vi "HB_OpenLog.vi"(8 "error in (no error)":errorcluster, 10 "File Name":string, 11 "“HBDeviceRef_in":T1) -> (0 "error out":errorcluster, 3 "“HBDeviceRef_out":T1)   [LabVIEW 2016]
uses:
  <vilib>/Rock Robotics/WPI/SerialPort/WPI_SerialPortRef.ctl
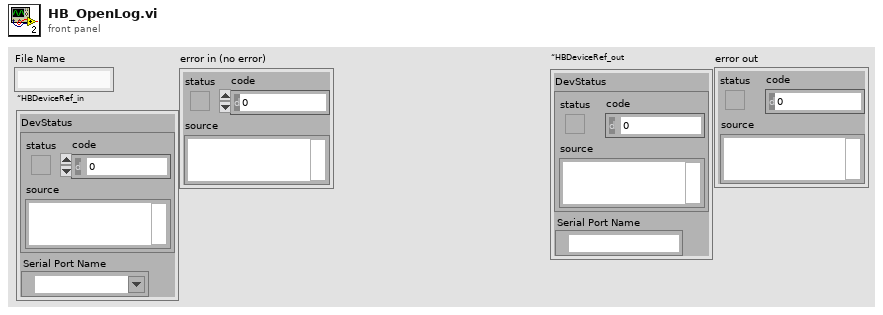
[diagram p1: front panel]
types:
  T1 = typedef "WPI_SerialPortRef.ctl" = cluster{"DevStatus":errorcluster, "Serial Port Name":refnum<visa-resource-name>}
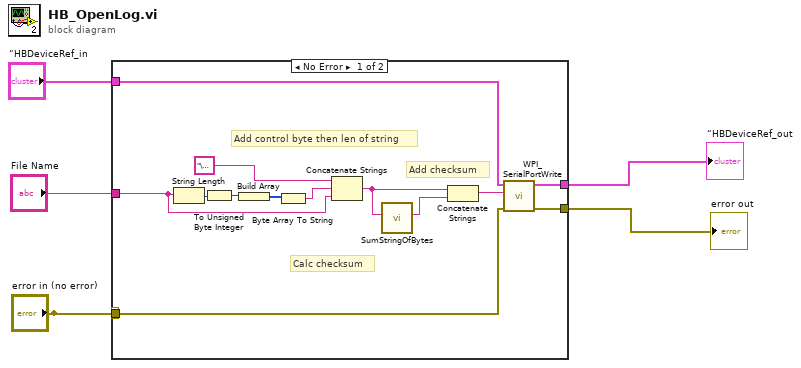
[diagram p0: block diagram]
diagram:
  n1 = case shown="No Error" "error in (no error)" {
    selector: "error in (no error)" -> [_ w19]
    tunnel: "File Name" -> [w10 _]
    tunnel: "“HBDeviceRef_in" -> [w9 w20]
    tunnel: [w8 w20] -> w3
    tunnel: "error in (no error)" -> [w7 _]
    tunnel: [w6 w19] -> w2
    frame No Error {
      # "Calc checksum"
      # "Add checksum"
      # "Add control byte then len of string"
      n2 = String Length(string=w10) -> (length=w12:i32)
      n3 = To Unsigned Byte Integer(number=w12) -> (unsigned 8bit integer=w15:u8)
      n4 = Build Array(w15) -> (w14:u8[])
      n5 = Byte Array To String(unsigned byte array=w14) -> (string=w13:string)
      n6 = Concatenate Strings("\u0003", w13, w10) -> (w17:string)
      n7 = call "SumStringOfBytes.vi"("String Of Bytes"=w17) -> ("SumAsString"=w18:string)  [unwired: 10 in]
      n8 = Concatenate Strings(w17, w18) -> (w11:string)
      n9 = call <vilib>:"WPI_SerialPortWrite.vi"("error in (no error)"=w7, "Buffer"=w11, "SerialPortRef"=w9) -> ("error out"=w6:errorcluster, "SerialPortRef"=w8:T1)  [unwired: 6 in, 1 out]
    }
    frame Error {
    }
  }
  "“HBDeviceRef_out" <- w3
  "error out" <- w2
